vi "Read Limit(Boolean).vi"(7 "Test":string, 8 "error in (no error)":errorcluster) -> (0 "error out":errorcluster, 2 "LowLimit":bool, 3 "HighLimit":bool)   [LabVIEW 2019, in "Unit Test Engine Tools.lvlib"]
uses:
  Unit Test Engine Tools.lvlib
  LVUT Global 1.vi
  <vilib>/Utility/file.llb/Read Delimited Spreadsheet (string).vi
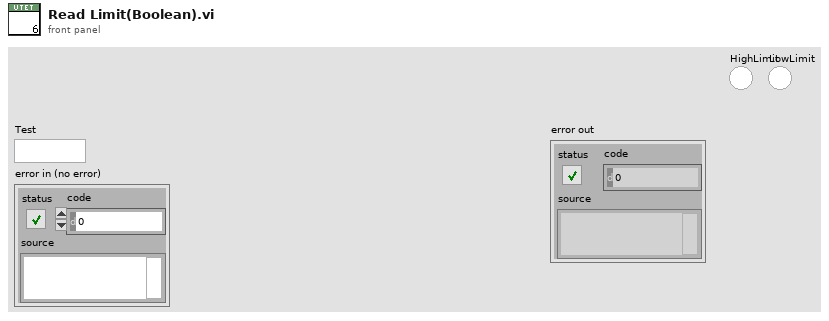
[diagram p1: front panel]
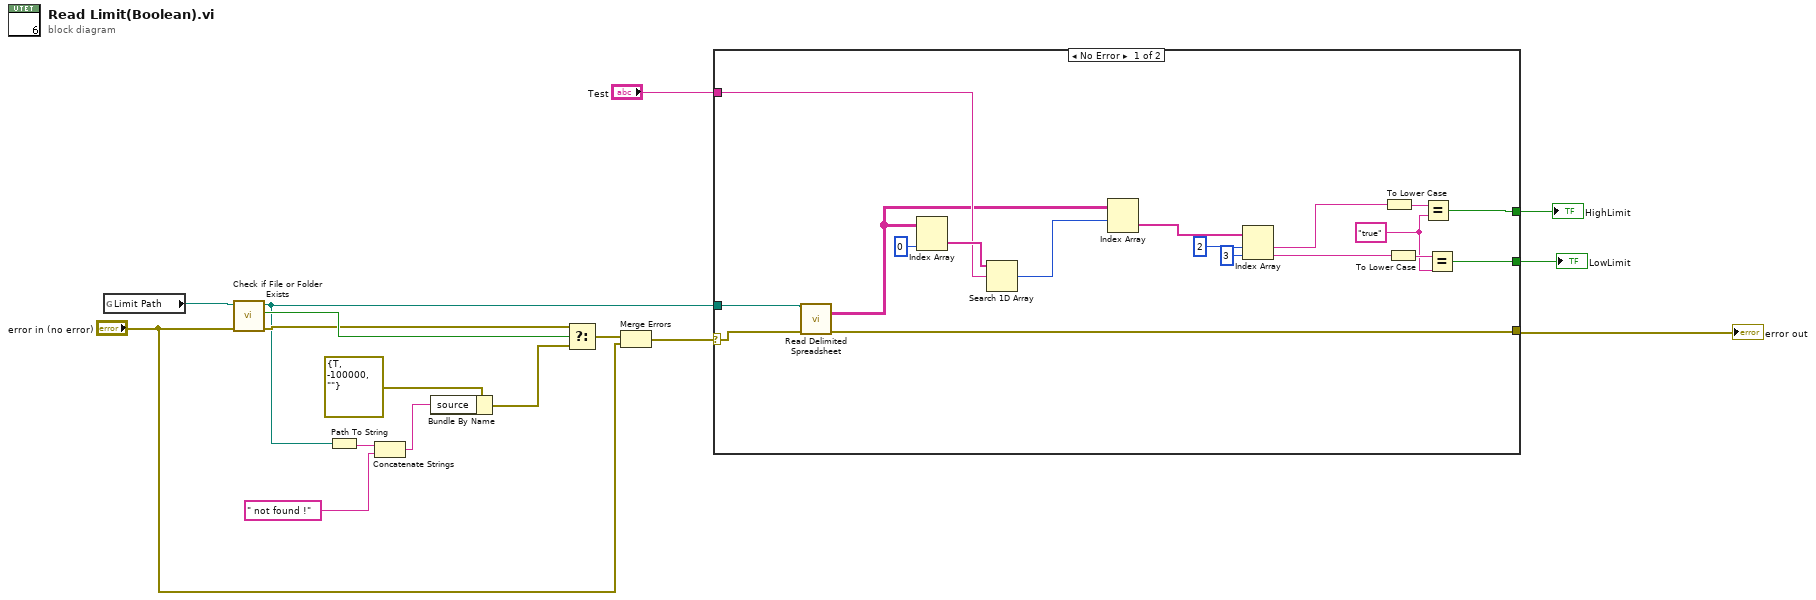
[diagram p0: block diagram]
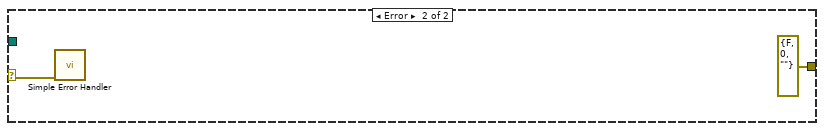
[diagram p2: hidden frame]
diagram:
  n1 = global read "LVUT Global 1.vi" "Limit Path"() -> (w10:path)
  n2 = call <vilib>:"Check if File or Folder Exists.vi"("error in (no error)"="error in (no error)", "path"=w10) -> ("error out"=w8:errorcluster, "file or folder exists?"=w9:bool, "dup path"=w2:path)  [unwired: 7 in]
  n3 = Path To String(path=w2) -> (string=w12:string)
  n4 = Concatenate Strings(w12, " not found !" ("string")) -> (w5:string)
  n5 = Bundle By Name(cluster=errorcluster {"status"=TRUE, "code"=-100000, "source"=""} ("f"), "source"=w5) -> (w6:errorcluster)
  n6 = Select(t=w8, s=w9, f=w6) -> (s? t:f=w4:errorcluster)
  n7 = Merge Errors(w4, "error in (no error)") -> (w3:errorcluster)
  n8 = case shown="No Error" w3 {
    selector: w3 -> [w18 w36]
    tunnel: "Test" -> [w29 _]
    tunnel: [w21 _] -> w15
    tunnel: [w20 _] -> w14
    tunnel: [w19 errorcluster {"status"=FALSE, "code"=0, "source"=""} ("error out")] -> w13
    tunnel: w2 -> [w17 _]
    frame No Error {
      w32 = "true" ("y")
      n9 = call-poly <vilib>:"Read Delimited Spreadsheet.vi"("file path (dialog if empty)"=w17, "error in (no error)"=w18) -> ("all rows"=w28:string[][], "error out"=w19:errorcluster)  [unwired: 8 in, 4 out]
      n10 = Index Array(array=w28, index (col)=0 ("disabled index (col)")) -> (element=w30:string[])  [unwired: 1 in]
      n11 = Search 1D Array(1D array=w30, element=w29) -> (index of element=w27:i32)  [unwired: 1 in]
      n12 = Index Array(array=w28, index (row)=w27) -> (element=w26:string[])  [unwired: 1 in]
      n13 = Index Array(array=w26, index #1=2 ("index"), index #2=3 ("index")) -> (element #1=w23:string, element #2=w22:string)
      n14 = To Lower Case(string=w23) -> (all lower case string=w34:string)
      n15 = To Lower Case(string=w22) -> (all lower case string=w33:string)
      n16 = Equal?(x=w34, y=w32) -> (x = y?=w21:bool)
      n17 = Equal?(x=w33, y=w32) -> (x = y?=w20:bool)
    }
    frame Error {
      n18 = call <vilib>:"Simple Error Handler.vi"("error in (no error)"=w36) -> ()  [unwired: 4 in, 5 out]
    }
  }
  "error out" <- w13
  "HighLimit" <- w15
  "LowLimit" <- w14
